vi "StartAsynchroneVi.vi"(7 "Open Front Panel ?":bool, 8 "error in":errorcluster, 9 "State":T1(ring), 10 "viInitString":string, 11 "viPathToStart":path) -> (0 "error out":errorcluster, 3 "vi reference":refnum<vi>)   [LabVIEW 2011]
uses:
  050 - CONFIG/00 - ApplicationConfig/Ctrls/EnumFgvConfigCommand.ctl
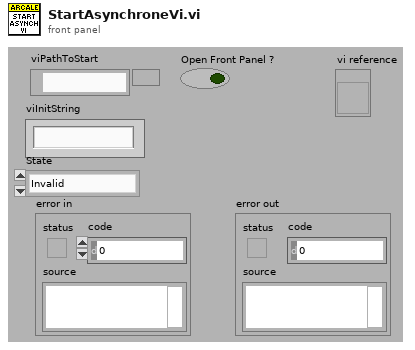
[diagram p1: front panel]
types:
  T1 = enum32{"Invalid", "Standard", "Closed", "Hidden", "Minimized", "Maximized"}
  T2 = enum32{"Bad", "Idle", "Run top level", "Running"}
  T3 = typedef "EnumFgvConfigCommand.ctl" = enum16{"Load", "Get", "Set", "Save To Disk"}
  T4 = typedef "ApplicationConfig.ctl" = cluster{"Data Path":path, "MessageHandlerConfig":T5, "Simulation":bool, "Dictionnary":string}
  T5 = typedef "MessageHandlerConfig.ctl" = cluster{"Max log files":u32, "Max messages per file":u32}
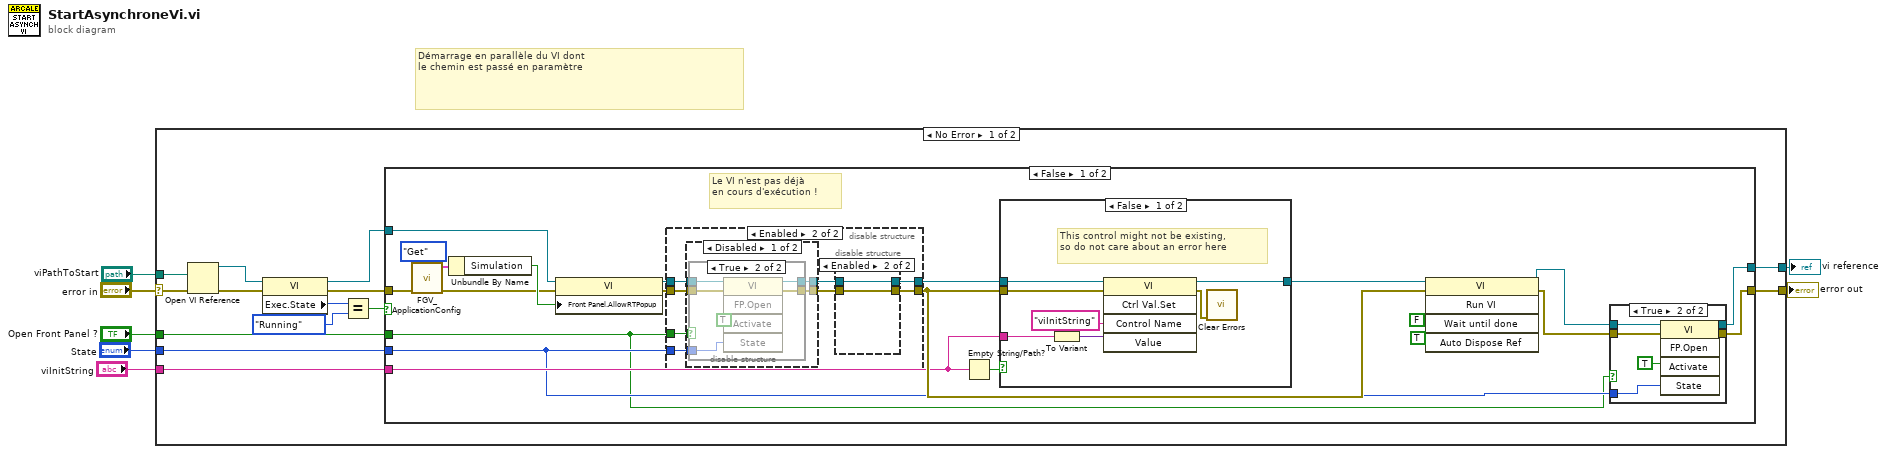
[diagram p0: block diagram]
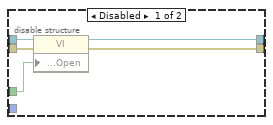
[diagram p4: hidden frame]
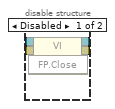
[diagram p5: hidden frame]
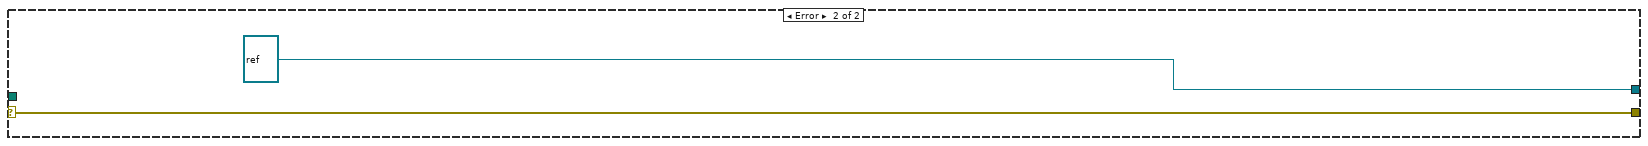
[diagram p9: hidden frame]
diagram:
  # "Démarrage en parallèle du VI dont\nle chemin est passé en paramètre"
  n1 = case shown="No Error" "error in" {
    selector: "error in" -> [w12 w97]
    tunnel: [w21 w97] -> w7
    tunnel: [w20 refnum<vi> refnum ("vi reference")] -> w6
    tunnel: "Open Front Panel ?" -> [w10 _]
    tunnel: "viPathToStart" -> [w11 _]
    tunnel: "viInitString" -> [w9 _]
    tunnel: "State" -> [w8 _]
    frame No Error {
      n2 = Open VI Reference(vi path=w11, error in (no error)=w12) -> (vi reference=w15:refnum<vi>, error out=w17:errorcluster)  [unwired: 1 in, 3 out]
      n3 = property class="VI"(reference=w15, error in=w17) -> (reference out=w14:refnum<vi>, error out=w16:errorcluster, "Exec.State"=w19:T2)
      n4 = Equal?(x=w19, y=T2."Running") -> (x = y?=w13:bool)
      n5 = case shown="False" w13 {
        tunnel: [w22 w95] -> w21
        tunnel: [w25 w94] -> w20
        tunnel: w16 -> [w40 w95]
        tunnel: w14 -> [w35 w94]
        tunnel: w10 -> [w23 _]
        tunnel: w9 -> [w28 _]
        tunnel: w8 -> [w24 _]
        frame False {
          # "Le VI n'est pas déjà\nen cours d'exécution !"
          n6 = call "FGV_ApplicationConfig.vi"("Command"=EnumFgvConfigCommand."Get", "error in (no error)"=w40) -> ("error out"=w36:errorcluster, "ApplicationConfigOut"=w38:T4)  [unwired: 8 in]
          n7 = Unbundle By Name(w38) -> ("Simulation"=w37:bool)
          n8 = property class="VI"(reference=w35, error in=w36, "Front Panel.AllowRTPopup"=w37) -> (reference out=w34:refnum<vi>, error out=w33:errorcluster)
          n9 = disable-structure shown="Enabled" {
            disable-tunnel: w34 -> [w63 w69]
            disable-tunnel: w33 -> [w62 w68]
            disable-tunnel: [w61 w71] -> w32
            disable-tunnel: [w60 w70] -> w30
            disable-tunnel: w23 -> [w59 w64]
            disable-tunnel: w24 -> [_ w65]
            frame Disabled {
              n10 = property class="VI"(reference=w63, error in=w62, "Front Panel Window:Open"=w59) -> (reference out=w61:refnum<vi>, error out=w60:errorcluster)
            }
            frame Enabled {
              n11 = disable-structure shown="Disabled" {
                disable-tunnel: w69 -> [w78 w93]
                disable-tunnel: w68 -> [w83 w92]
                disable-tunnel: [w82 w92] -> w67
                disable-tunnel: [w79 w93] -> w66
                disable-tunnel: w65 -> [w81 _]
                disable-tunnel: w64 -> [w80 _]
                frame Disabled {
                  n12 = case shown="True" w80 {
                    tunnel: _ -> [w85 _]
                    tunnel: w83 -> [w84 w91]
                    tunnel: [w84 w90] -> w82
                    tunnel: [w85 w89] -> w79
                    tunnel: w81 -> [_ w87]
                    tunnel: w78 -> [_ w86]
                    frame False {
                    }
                    frame True {
                      n13 = invoke class="VI" method="FP.Open"(reference=w86, error in=w91, "Activate"=TRUE ("Activate?"), "State"=w87) -> (reference out=w89:refnum<vi>, error out=w90:errorcluster)  [unwired: 1 in, 3 out]
                    }
                  }
                }
                frame Enabled {
                }
              }
              n14 = disable-structure shown="Enabled" {
                disable-tunnel: [w75 w77] -> w71
                disable-tunnel: [w74 w76] -> w70
                disable-tunnel: w67 -> [w73 w76]
                disable-tunnel: w66 -> [w72 w77]
                frame Disabled {
                  n15 = invoke class="VI" method="FP.Close"(reference=w72, error in=w73) -> (reference out=w75:refnum<vi>, error out=w74:errorcluster)  [unwired: 1 in, 1 out]
                }
                frame Enabled {
                }
              }
            }
          }
          n16 = Empty String/Path?(string/path=w28) -> (empty?=w29:bool)
          n17 = case shown="False" w29 {
            tunnel: w32 -> [w57 w58]
            tunnel: [w56 w58] -> w31
            tunnel: w30 -> [w53 _]
            tunnel: w28 -> [w51 _]
            frame False {
              # "This control might not be existing,\nso do not care about an error here"
              n18 = To Variant(anything=w51) -> (Variant=w52:variant)
              n19 = invoke class="VI" method="Ctrl Val.Set"(reference=w57, error in=w53, "Control Name"="viInitString", "Value"=w52) -> (reference out=w56:refnum<vi>, error out=w54:errorcluster)  [unwired: 1 in, 3 out]
              n20 = call <vilib>:"Clear Errors.vi"("error in (no error)"=w54) -> ()  [unwired: 6 in, 1 out]
            }
            frame True {
            }
          }
          n21 = invoke class="VI" method="Run VI"(reference=w31, error in=w30, "Wait until done"=FALSE ("Wait Until Done"), "Auto Dispose Ref"=TRUE ("Auto Dispose Reference")) -> (reference out=w26:refnum<vi>, error out=w27:errorcluster)  [unwired: 1 in, 3 out]
          n22 = case shown="True" w23 {
            tunnel: w26 -> [w44 w50]
            tunnel: w27 -> [w43 w49]
            tunnel: [w43 w48] -> w22
            tunnel: [w44 w47] -> w25
            tunnel: w24 -> [_ w45]
            frame False {
            }
            frame True {
              n23 = invoke class="VI" method="FP.Open"(reference=w50, error in=w49, "Activate"=TRUE ("Activate?"), "State"=w45) -> (reference out=w47:refnum<vi>, error out=w48:errorcluster)  [unwired: 1 in, 3 out]
            }
          }
        }
        frame True {
        }
      }
    }
    frame Error {
    }
  }
  "error out" <- w7
  "vi reference" <- w6
